vi "get_file_info.vi"(8 "error in (no error)":errorcluster, 11 "File Path in":path) -> (0 "error out":errorcluster, 2 "String Times":T3, 3 "File Path out":path)   [LabVIEW 2010, in "TrajectoryMH100122AODRAPS.lvclass"]
uses:
  TrajectoryMH100122AODRAPS.lvclass
  kernel32.dll
panel:
  out "Creation Time":T1={"Year"=0, "Month"=1, "DayOfWeek"=0, "Day"=0, "Hour"=0, "Minute"=0, "Seconds"=0, "Milliseconds"=0} {"DayOfWeek" items=["Sunday", "Monday", "Tuesday", "Wednesday", "Thursday", "Friday", "Saturday"]; "Month" items=["", "January", "February", "March", "April", "May", "June", "July", "August", "September", "October", "November", "December"]}
  out "Last Access Time":T1={"Year"=0, "Month"=1, "DayOfWeek"=0, "Day"=0, "Hour"=0, "Minute"=0, "Seconds"=0, "Milliseconds"=0} {"DayOfWeek" items=["Sunday", "Monday", "Tuesday", "Wednesday", "Thursday", "Friday", "Saturday"]; "Month" items=["", "January", "February", "March", "April", "May", "June", "July", "August", "September", "October", "November", "December"]}
  out "Last Write Time":T1={"Year"=0, "Month"=1, "DayOfWeek"=0, "Day"=0, "Hour"=0, "Minute"=0, "Seconds"=0, "Milliseconds"=0} {"DayOfWeek" items=["Sunday", "Monday", "Tuesday", "Wednesday", "Thursday", "Friday", "Saturday"]; "Month" items=["", "January", "February", "March", "April", "May", "June", "July", "August", "September", "October", "November", "December"]}
  out "File Attributes":T2
  out "File size (bytes)":string
  in  "Time Format String (%c)":string="%c"
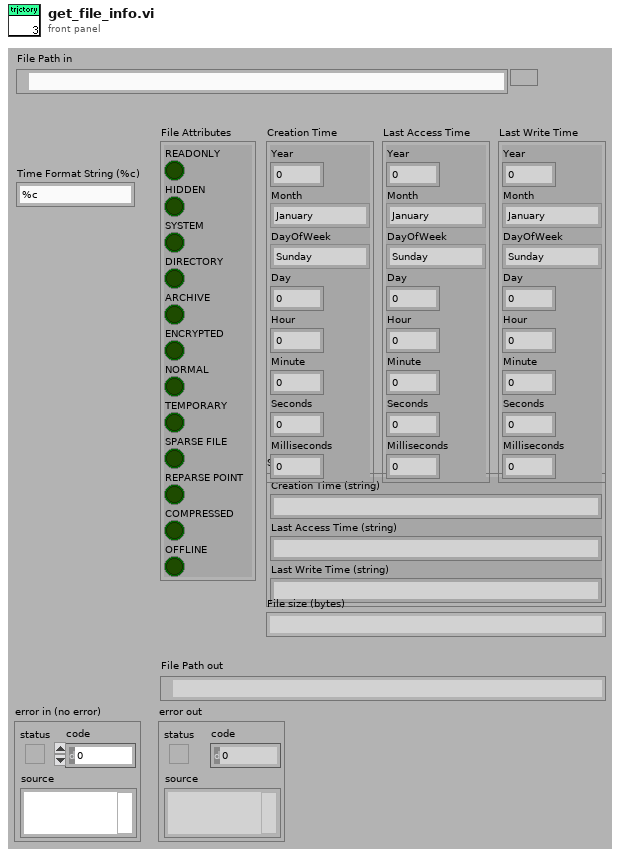
[diagram p1: front panel]
types:
  T1 = cluster{"Year":u16, "Month":u16, "DayOfWeek":u16, "Day":u16, "Hour":u16, "Minute":u16, "Seconds":u16, "Milliseconds":u16}
  T2 = cluster{"READONLY":bool, "HIDDEN":bool, "SYSTEM":bool, "DIRECTORY":bool, "ARCHIVE":bool, "ENCRYPTED":bool, "NORMAL":bool, "TEMPORARY":bool, "SPARSE FILE":bool, "REPARSE POINT":bool, "COMPRESSED":bool, "OFFLINE":bool}
  T3 = cluster{"Creation Time (string)":string, "Last Access Time (string)":string, "Last Write Time (string)":string}
  T4 = cluster{"wYear":u16, "wMonth":u16, "wDayOfWeek":u16, "wDay":u16, "wHour":u16, "wMinute":u16, "wSeconds":u16, "wMilliseconds 2":u16}
  T5 = cluster{"dwFileAttributes":u32, "ftCreationTime":cluster{"dwLowDateTime":i32, "dwHighDateTime":i32}, "ftLastAccessTime":cluster{"dwLowDateTime":i32, "dwHighDateTime":i32}, "ftLastWriteTime":cluster{"dwLowDateTime":i32, "dwHighDateTime":i32}, "nFileSizeHigh":u32, "nFileSizeLow":u32}
  T6 = cluster{"dwLowDateTime":i32, "dwHighDateTime":i32}
  T7 = cluster{"[0]":bool, "[1]":bool, "[2]":bool, "[3]":bool, "[4]":bool, "[5]":bool, "[6]":bool, "[7]":bool, "[8]":bool, "[9]":bool, "[10]":bool, "[11]":bool}
  T8 = cluster{"UTC Date and Time out (string)":string, "UTC Date and Time out (string)":string, "UTC Date and Time out (string)":string}
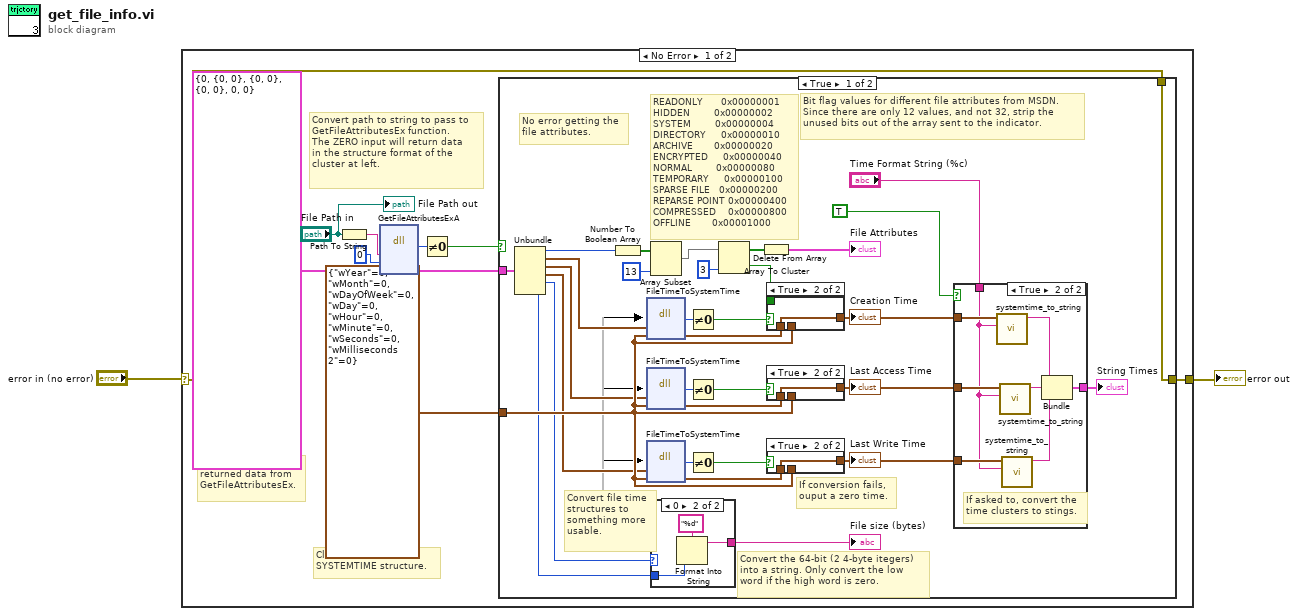
[diagram p0: block diagram]
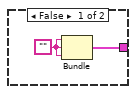
[diagram p2: hidden frame]
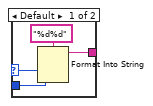
[diagram p3: hidden frame]
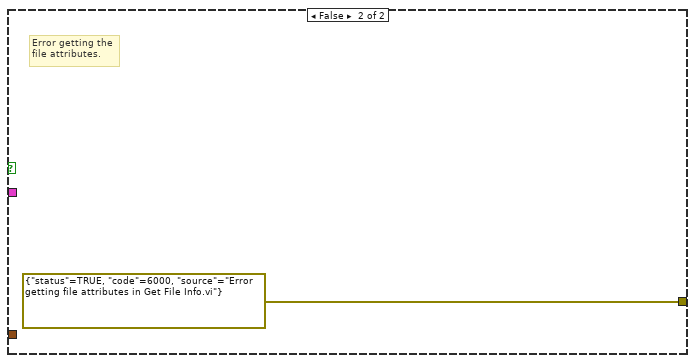
[diagram p7: hidden frame]
diagram:
  n1 = case shown="No Error" "error in (no error)" {
    selector: "error in (no error)" -> [w3 w69]
    tunnel: [w4 w69] -> w2
    frame No Error {
      # "Convert path to string to pass to\nGetFileAttributesEx function.\nThe ZERO input will return data\nin the structure format of the\ncluster at left."
      # "Cluster constant for\nSYSTEMTIME structure."
      # "Cluster constant for\nreturned data from\nGetFileAttributesEx."
      n2 = Path To String(path="File Path in") -> (string=w10:string)
      n3 = dll-call lib="KERNEL32.DLL" fn="GetFileAttributesExA" label="GetFileAttributesEx"("lpFileName"=w10, "fInfoLevelID"=0, T5 {"dwFileAttributes"=0, "ftCreationTime"={"dwLowDateTime"=0, "dwHighDateTime"=0}, "ftLastAccessTime"={"dwLowDateTime"=0, "dwHighDateTime"=0}, "ftLastWriteTime"={"dwLowDateTime"=0, "dwHighDateTime"=0}, "nFileSizeHigh"=0, "nFileSizeLow"=0}) -> (w9:i32, w6:T5)  [unwired: 5 in, 2 out]
      n4 = Not Equal To 0?(x=w9) -> (x != 0?=w5:bool)
      n5 = case shown="True" w5 {
        tunnel: T4 {"wYear"=0, "wMonth"=0, "wDayOfWeek"=0, "wDay"=0, "wHour"=0, "wMinute"=0, "wSeconds"=0, "wMilliseconds 2"=0} -> [w35 _]
        tunnel: w6 -> [w21 _]
        tunnel: [w13 errorcluster {"status"=TRUE, "code"=6000, "source"="Error getting file attributes in Get File Info.vi"} ("error out")] -> w4
        tunnel: w3 -> [w13 _]
        frame True {
          # "If conversion fails,\nouput a zero time."
          # "Convert the 64-bit (2 4-byte itegers)\ninto a string. Only convert the low\nword if the high word is zero."
          # "Convert file time\nstructures to\nsomething more\nusable."
          # "Bit flag values for different file attributes from MSDN.\nSince there are only 12 values, and not 32, strip the\nunused bits out of the array sent to the indicator."
          # "No error getting the\nfile attributes."
          # "READONLY      0x00000001\nHIDDEN        0x00000002\nSYSTEM        0x00000004\nDIRECTORY     0x00000010\nARCHIVE       0x00000020\nENCRYPTED     0x00000040\nNORMAL        0x00000080\nTEMPORARY     0x00000100\nSPARSE FILE   0x00000200\nREPARSE POINT 0x00000400\nCOMPRESSED    0x00000800\nOFFLINE       0x00001000"
          n6 = Unbundle(w21) -> ("dwFileAttributes"=w26:u32, "ftCreationTime"=w20:T6, "ftLastAccessTime"=w22:T6, "ftLastWriteTime"=w23:T6, "nFileSizeHigh"=w24:u32, "nFileSizeLow"=w25:u32)
          n7 = Number To Boolean Array(number=w26) -> (Boolean array=w34:bool[])
          n8 = dll-call lib="KERNEL32.DLL" fn="FileTimeToSystemTime"("ftCreationTime"=w20, w35) -> (w44:i32, w40:T4)  [unwired: 4 in, 2 out]
          n9 = dll-call lib="KERNEL32.DLL" fn="FileTimeToSystemTime"("ftLastAccessTime"=w22, w35) -> (w43:i32, w38:T4)  [unwired: 4 in, 2 out]
          n10 = dll-call lib="KERNEL32.DLL" fn="FileTimeToSystemTime"("ftLastWriteTime"=w23, w35) -> (w42:i32, w36:T4)  [unwired: 4 in, 2 out]
          n11 = Array Subset(array=w34, length=13) -> (w32:bool[])  [unwired: 1 in]
          n12 = case shown="0" w24 {
            selector: w24 -> [w55 _]
            tunnel: w25 -> [w58 w61]
            tunnel: [w56 w59] -> w27
            frame Default {
              n13 = Format Into String(format string="%d%d", w55, w58) -> (resulting string=w56:string)  [unwired: 2 in, 1 out]
            }
            frame 0 {
              n14 = Format Into String(format string="%d", w61) -> (resulting string=w59:string)  [unwired: 2 in, 1 out]
            }
          }
          "File size (bytes)" <- w27
          n15 = Not Equal To 0?(x=w44) -> (x != 0?=w41:bool)
          n16 = Not Equal To 0?(x=w43) -> (x != 0?=w39:bool)
          n17 = Not Equal To 0?(x=w42) -> (x != 0?=w37:bool)
          n18 = Delete From Array(array=w32, index=3) -> (deleted portion=w30:bool, array with subset deleted=w29:bool[])  [unwired: 1 in]
          n19 = Array To Cluster(array=w29) -> (cluster=→"File Attributes":T7)
          n20 = case shown="True" w41 {
            tunnel: w40 -> [_ w67]
            tunnel: w35 -> [w66 _]
            tunnel: [w66 w67] -> w18
            tunnel: w30 -> [_ _]
            frame False {
            }
            frame True {
            }
          }
          "Creation Time" <- w18
          n21 = case shown="True" w39 {
            tunnel: w38 -> [_ w65]
            tunnel: w35 -> [w64 _]
            tunnel: [w64 w65] -> w17
            frame False {
            }
            frame True {
            }
          }
          "Last Access Time" <- w17
          n22 = case shown="True" w37 {
            tunnel: w36 -> [_ w63]
            tunnel: w35 -> [w62 _]
            tunnel: [w62 w63] -> w16
            frame False {
            }
            frame True {
            }
          }
          "Last Write Time" <- w16
          n23 = case shown="True" TRUE ("Convert times to string? (F)") {
            tunnel: w18 -> [_ w53]
            tunnel: w17 -> [_ w50]
            tunnel: w16 -> [_ w51]
            tunnel: "Time Format String (%c)" -> [_ w49]
            tunnel: [w46 w54] -> w14
            frame False {
              w45 = ""
              n24 = Bundle(w45, w45, w45) -> (w46:cluster{string, string, string})  [unwired: 1 in]
            }
            frame True {
              # "If asked to, convert the\ntime clusters to stings."
              n25 = call "systemtime_to_string.vi"("time format string (%c)"=w49, "UTC Date and Time in"=w53) -> ("UTC Date and Time out (string)"=w52:string)  [unwired: 9 in]
              n26 = call "systemtime_to_string.vi"("time format string (%c)"=w49, "UTC Date and Time in"=w50) -> ("UTC Date and Time out (string)"=w47:string)  [unwired: 9 in]
              n27 = call "systemtime_to_string.vi"("time format string (%c)"=w49, "UTC Date and Time in"=w51) -> ("UTC Date and Time out (string)"=w48:string)  [unwired: 9 in]
              n28 = Bundle("UTC Date and Time out (string)"=w52, "UTC Date and Time out (string)"=w47, "UTC Date and Time out (string)"=w48) -> (w54:T8)  [unwired: 1 in]
            }
          }
          "String Times" <- w14
        }
        frame False {
          # "Error getting the\nfile attributes."
        }
      }
      "File Path out" <- "File Path in"
    }
    frame Error {
      # "Since there was an error before we begin this\nVI, do nothing and pass the error though."
    }
  }
  "error out" <- w2
